vi "Acquire.vi"(7 "Signal Type":T1, 8 "error in (no error)":errorcluster, 10 "Rate":dbl=1.0, 11 "HW ID in":string="Dev0/Ti0:7") -> (0 "error out":errorcluster, 2 "Graph Data":waveform(dbl)[](array[waveform])=[{"t0"=timestamp(3726699625.76544 s since 1904-01-01), "dt"=1.0, "Y"=[270.1504414462806]}, {"t0"=timestamp(3726699625.76544 s since 1904-01-01), "dt"=1.0, "Y"=[271.2700685989695]}, {"t0"=timestamp(3726699625.76544 s since 1904-01-01), "dt"=1.0, "Y"=[272.92783695695294]}], 3 "HW ID out":string)   [LabVIEW 2019, in "Acquisition.lvlib"]
doc: "Perform the acquisition. Replace the contents of this diagram with calls to acquisition hardware.\n_____\nBased on DQMH Project Template 6.0.0.91."
uses:
  Acquisition.lvlib
  CML Shared/Signal Type--enum.ctl
  <vilib>/ULx/Read.llb/ULx Read (Analog 1D DBL NChan 1Samp).vi
  <vilib>/ULx/Create Channel.llb/ULx Create Channel (AI-Temperature).vi
  CML Shared/CML Shared.lvlib
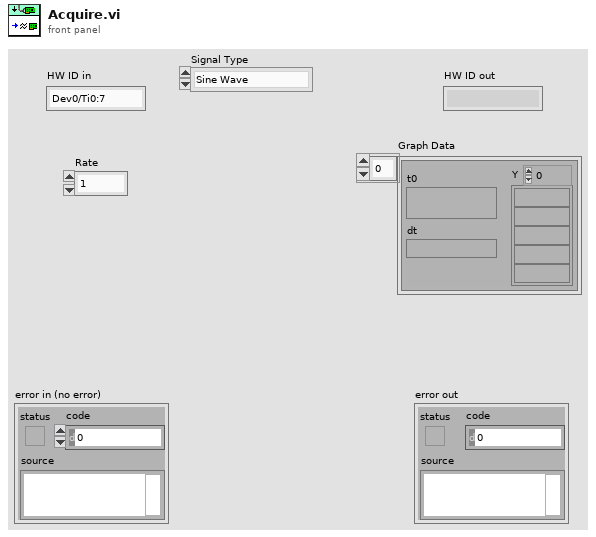
[diagram p1: front panel]
types:
  T1 = typedef "CML Shared.lvlib/Signal Type--enum.ctl" = enum16{"Sine Wave", "Square with Noise"}
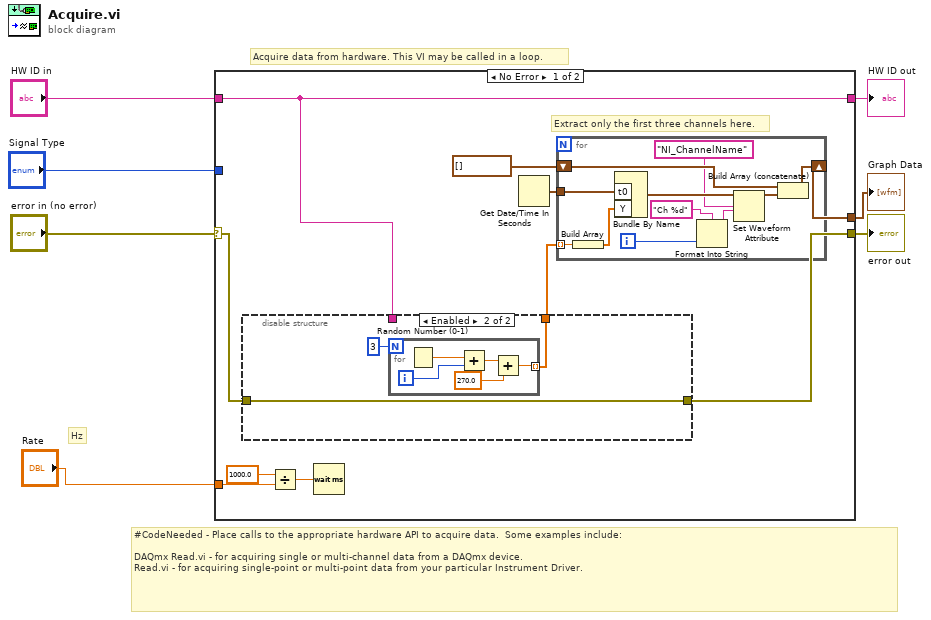
[diagram p0: block diagram]
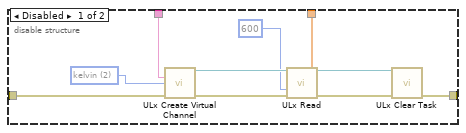
[diagram p2: hidden frame]
diagram:
  # "Hz"
  # "Acquire data from hardware. This VI may be called in a loop."
  # "#CodeNeeded - Place calls to the appropriate hardware API to acquire data.  Some examples include:\n\nDAQmx Read.vi - for acquiring single or multi-channel data from a DAQmx device.\nRead.vi - for acquiring single-point or multi-point data from your particular Instrument Driver."
  n1 = case shown="No Error" "error in (no error)" {
    selector: "error in (no error)" -> [w12 w47]
    tunnel: [w13 w47] -> w6
    tunnel: "HW ID in" -> [w11 w48]
    tunnel: [w11 w48] -> w4
    tunnel: "Signal Type" -> [_ _]
    tunnel: [w15 _] -> w2
    tunnel: "Rate" -> [w9 _]
    frame No Error {
      # "Extract only the first three channels here."
      n2 = disable-structure shown="Enabled" {
        disable-tunnel: [w22 w30] -> w13
        disable-tunnel: w12 -> [w21 w30]
        disable-tunnel: [w19 w28] -> w14
        disable-tunnel: w11 -> [w18 _]
        frame Disabled {
          w20 = 2 items=["degC", "degF", "kelvin", "raw"] ("units")
          n3 = call-poly <vilib>:"ULx Create Virtual Channel.vi"("physical channels"=w18, "units"=w20, "error in"=w21) -> ("task out"=w26:refnum<k24>, "error out"=w27:errorcluster)  [unwired: 11 in]
          n4 = call-poly <vilib>:"ULx Read.vi"("task in"=w26, "timeout"=600, "error in"=w27) -> ("task out"=w25:refnum<k24>, "data"=w19:dbl[], "error out"=w24:errorcluster)  [unwired: 10 in]
          n5 = call <vilib>:"ULx Clear Task.vi"("task in"=w25, "error in"=w24) -> ("error out"=w22:errorcluster)  [unwired: 13 in]
        }
        frame Enabled {
          n6 = for {
            N: 3 -> [_]
            tunnel: [w33] -> w28 mode=indexing
            i -> [w34]
            n7 = Random Number (0-1)() -> (number: 0 to 1=w35:dbl)
            n8 = Add(x=w35, y=w34) -> (x+y=w32:dbl)
            n9 = Add(x=w32, y=270.0) -> (x+y=w33:dbl)
          }
        }
      }
      n10 = Divide(x=1000.0, y=w9) -> (x/y=w10:dbl)
      n11 = Wait (ms)(milliseconds to wait=w10) -> ()  [unwired: 1 out]
      n12 = Get Date/Time In Seconds() -> (seconds since 1Jan1904=w17:timestamp)
      n13 = for {
        tunnel: w17 -> [w46]
        tunnel: w14 -> [w45] mode=indexing
        shift-right: [w43] -> w15
        shift-left: waveform(dbl)[] [] -> [w42]
        i -> [w36]
        n14 = Build Array(w45) -> (w44:dbl[])
        n15 = Bundle By Name("t0"=w46, "Y"=w44) -> (w40:waveform(dbl))  [unwired: 1 in]
        n16 = Format Into String(format string="Ch %d", w36) -> (resulting string=w38:string)  [unwired: 2 in, 1 out]
        n17 = Set Waveform Attribute(5:w38, 6:"NI_ChannelName" ("name"), 7:w40) -> (3:w41:waveform(dbl))  [unwired: 1 in, 2 out]
        n18 = Build Array (concatenate)(w42, w41) -> (w43:waveform(dbl)[])
      }
    }
    frame Error {
    }
  }
  "HW ID out" <- w4
  "error out" <- w6
  "Graph Data" <- w2
